vi "队列主vi.vi"() -> ()   [LabVIEW 2024]
panel:
  in  "开始录音":bool
  in  "播放声音":bool
  in  "停止":bool
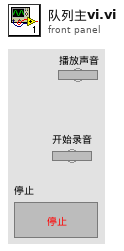
[diagram p1: front panel]
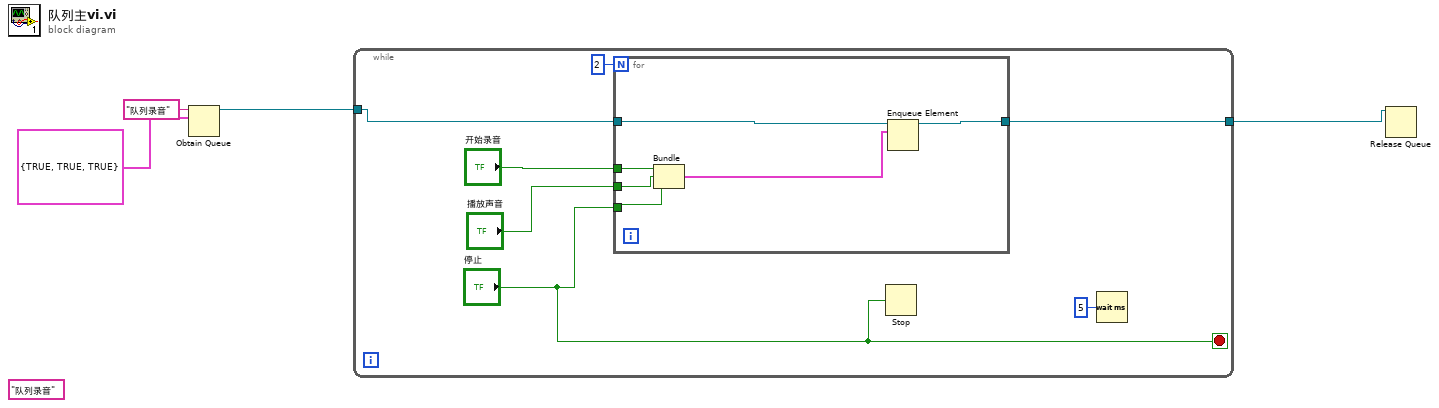
[diagram p0: block diagram]
diagram:
  (unwired) "队列录音" ("名称（未命名）")
  n1 = Obtain Queue(name (unnamed)="队列录音" ("名称（未命名）"), element data type=cluster{bool, bool, bool} {TRUE, TRUE, TRUE}) -> (queue out=w1:refnum<queue>)  [unwired: 3 in, 2 out]
  n2 = while {
    tunnel: w1 -> [w11]
    tunnel: [w10] -> w4
    stop <- "停止" stop-if-true
    n3 = for {
      N: 2 -> [_]
      tunnel: w11 -> [w17]
      tunnel: [w16] -> w10
      tunnel: "开始录音" -> [w15]
      tunnel: "播放声音" -> [w14]
      tunnel: "停止" -> [w13]
      n4 = Bundle("开始录音"=w15, "播放声音"=w14, "停止"=w13) -> (w12:cluster{"开始录音":bool, "播放声音":bool, "停止":bool})  [unwired: 1 in]
      n5 = Enqueue Element(queue=w17, element=w12) -> (queue out=w16:refnum<queue>)  [unwired: 2 in, 2 out]
    }
    n6 = Stop(stop? (T)="停止") -> ()
    n7 = Wait (ms)(milliseconds to wait=u32 5 ("等待时间（毫秒）")) -> ()  [unwired: 1 out]
  }
  n8 = Release Queue(queue=w4) -> ()  [unwired: 2 in, 3 out]
